vi "example_set_device_output_single.vi"() -> ()   [LabVIEW 2012]
doc: "EXAMPLE: Set Device Digital Output (single only)\n\nThis VI sets the value of one digital output channel at a time. Simply select the appropriate channel, select the output value (true or false) and run the VI!\n\nProduced By:\n\nChristopher Lemieux\nKod Integrations, LLC\n4835 Marianne Drive\nMount Airy, MD 21771\nhttp://www.kodintegrations.com\nemail: clemieux@kodintegrations.com\nphone: (240) 687-1288"
uses:
  support/controls/digital_output_items.ctl
panel:
  out "response":string
  in  "value":bool
  in  "digital_output":T1
  in  "device_index (def=0)":i32
  out "error out":errorcluster
  in  "error in (no error)":errorcluster
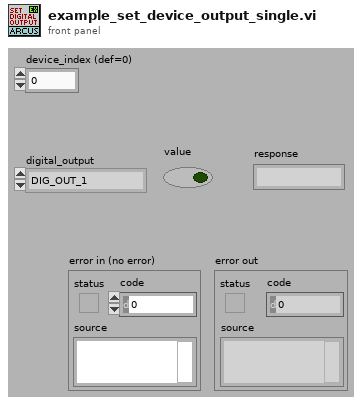
[diagram p1: front panel]
types:
  T1 = typedef "digital_output_items.ctl" = enum16{"DIG_OUT_1", "DIG_OUT_2"}
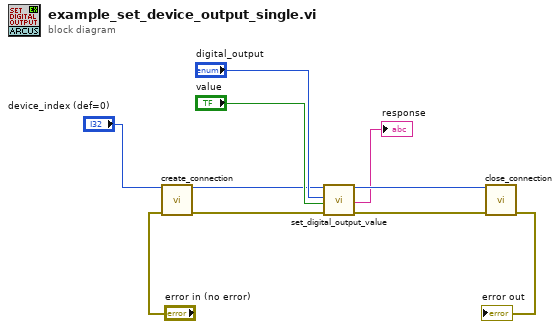
[diagram p0: block diagram]
diagram:
  n1 = call "create_connection.vi"("device_index (def=0)"="device_index (def=0)", "error in (no error)"="error in (no error)") -> ("reference"=w3:i32, "error out"=w2:errorcluster)  [unwired: 12 in]
  n2 = call "set_digital_output_value.vi"("reference (in)"=w3, "digital_output_ch"="digital_output", "dig_out_value"="value", "error in (no error)"=w2) -> ("reference (dup)"=w7:i32, "response"=→"response":string, "error out"=w6:errorcluster)  [unwired: 13 in]
  n3 = call "close_connection.vi"("reference"=w7, "error in (no error)"=w6) -> ("error out"=→"error out":errorcluster)  [unwired: 13 in]
